vi "Parse Build-in Error Codes.vi"(8 "error in (no error)":errorcluster, 11 "errors file content":string) -> (0 "error out":errorcluster, 1 "errors":T2[](array[typedef]), 2 "comment":string, 3 "family":T1)   [LabVIEW 2017, in "Error File Management.lvlib"]
uses:
  Error File Management.lvlib
  Controls/NI Error.ctl
  Controls/NI Family.ctl
  <vilib>/regexp/Match Regular Expression.xnode
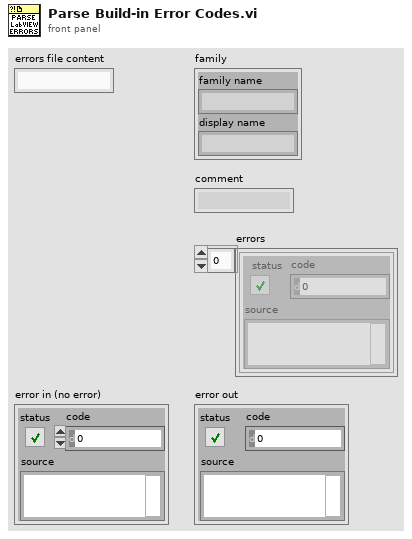
[diagram p1: front panel]
types:
  T1 = typedef "Error File Management.lvlib/NI Family.ctl" = cluster{"family name":string, "display name":string}
  T2 = typedef "Error File Management.lvlib/NI Error.ctl" = errorcluster
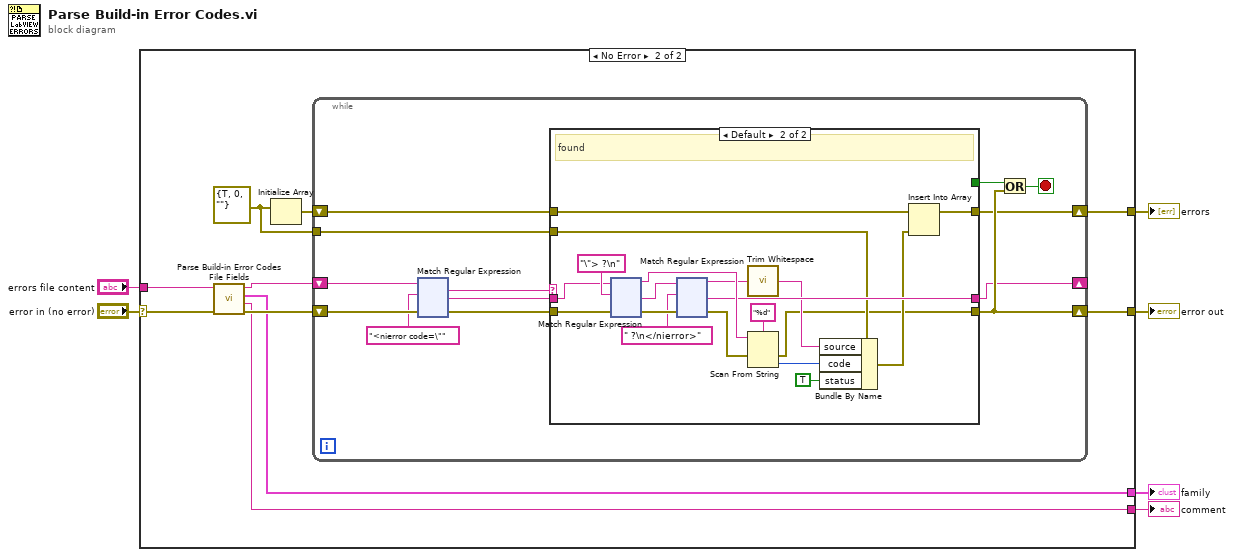
[diagram p0: block diagram]
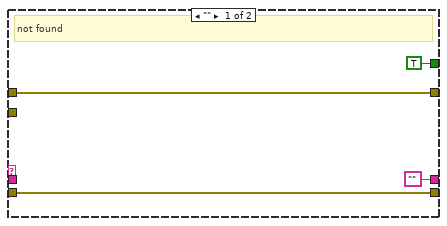
[diagram p3: hidden frame]
diagram:
  n1 = case shown="No Error" "error in (no error)" {
    selector: "error in (no error)" -> [w7 w14]
    tunnel: "errors file content" -> [_ w11]
    tunnel: [_ w17] -> w4
    tunnel: [w7 w15] -> w6
    tunnel: [_ w9] -> w2
    tunnel: [_ w8] -> w1
    frame Error {
    }
    frame No Error {
      w13 = T2 {"status"=TRUE, "code"=0, "source"=""} ("error")
      n2 = call "Parse Build-in Error Codes File Fields.vi"("error in (no error)"=w14, "errors file content in"=w11) -> ("error out"=w12:errorcluster, "comment"=w8:string, "family"=w9:T1, "errors file content dup"=w10:string)  [unwired: 6 in]
      n3 = Initialize Array(w13) -> (w16:T2[])  [unwired: 1 in]
      n4 = while {
        shift-right: [w26] -> _
        shift-left: w10 -> [w22]
        tunnel: w13 -> [w25]
        shift-right: [w23] -> w17
        shift-left: w16 -> [w24]
        shift-right: [w30] -> w15
        shift-left: w12 -> [w29]
        stop <- w18 stop-if-true
        n5 = xnode "Match Regular Expression"("input string"=w22, "regular expression"="<nierror code=\"", "error in"=w29) -> ("whole match"=w21:string, "after match"=w27:string, "error out"=w20:errorcluster)  [unwired: 3 in, 2 out]
        n6 = case shown="Default" w21 {
          tunnel: ["" w162] -> w26
          tunnel: w25 -> [_ w161]
          tunnel: w24 -> [w147 w160]
          tunnel: [w147 w159] -> w23
          tunnel: w27 -> [_ w156]
          tunnel: [TRUE _] -> w19
          tunnel: w20 -> [w146 w154]
          tunnel: [w146 w150] -> w30
          frame "" {
            # "not found"
          }
          frame Default {
            # "found"
            n7 = xnode "Match Regular Expression"("input string"=w156, "regular expression"="\"> ?\n", "error in"=w154) -> ("before match"=w163:string, "after match"=w155:string, "error out"=w167:errorcluster)  [unwired: 3 in, 2 out]
            n8 = xnode "Match Regular Expression"("input string"=w155, "regular expression"=" ?\n</nierror>", "error in"=w167) -> ("before match"=w158:string, "after match"=w162:string, "error out"=w153:errorcluster)  [unwired: 3 in, 2 out]
            n9 = call <vilib>:"Trim Whitespace.vi"("string"=w158) -> ("trimmed string"=w157:string)  [unwired: 1 in]
            n10 = Scan From String(format string="%d", input string=w163, error in=w153) -> (error out=w150:errorcluster, output 1=w152:i32)  [unwired: 2 in, 2 out]
            n11 = Bundle By Name(cluster=w161, "source"=w157, "code"=w152, "status"=TRUE) -> (w151:T2)
            n12 = Insert Into Array(array=w160, new element=w151) -> (w159:T2[])  [unwired: 1 in]
          }
        }
        n13 = Or(x=w19, y=w30) -> (x .or. y?=w18:bool)
      }
    }
  }
  "error out" <- w6
  "errors" <- w4
  "family" <- w2
  "comment" <- w1
